vi "matrixManipulation.vi"(10 "J Index":i32, 11 "Input Array":dbl[][](array[numeric])) -> (2 "Frequency Num":string, 3 "Output Array at Frequency Num":dbl[][](array[numeric]))   [LabVIEW 2012]
uses:
  <vilib>/Analysis/Matrix/Numeric/Conversions/Array To Matrix - RA2.vi
  <vilib>/Analysis/Matrix/Numeric/Conversions/Matrix To Array - RM.vi
  <vilib>/Analysis/Matrix/NI_Matrix.lvlib
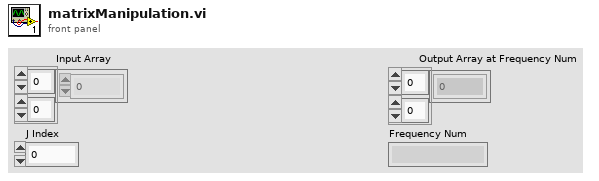
[diagram p1: front panel]
types:
  T1 = typedef "NI_Matrix.lvlib/RealMatrix.ctl" = dbl[][]
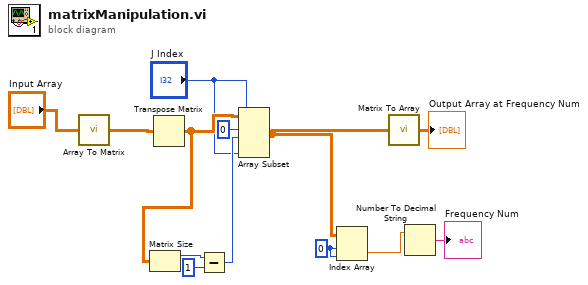
[diagram p0: block diagram]
diagram:
  w4 = 0 ("index (row)")
  n1 = call-poly <vilib>:"Array To Matrix.vi"("Real 2D Array"="Input Array") -> ("Real Matrix"=w12:T1)
  n2 = Transpose Matrix(1:w12) -> (0:w10:T1)
  n3 = Matrix Size(0:w10) -> (1:w9:i32)  [unwired: 1 out]
  n4 = Subtract(x=w9, y=1) -> (x-y=w7:i32)
  n5 = Array Subset(array=w10, index (row)=0 ("row 1"), length (row)=w7, index (col)="J Index", length (col)="J Index") -> (w1:T1)
  n6 = Index Array(array=w1, index (row)=w4, index (col)=w4) -> (element=w3:dbl)
  n7 = call-poly <vilib>:"Matrix To Array.vi"("Real Matrix"=w1) -> ("Real 2D Array"=→"Output Array at Frequency Num":dbl[][])
  n8 = Number To Decimal String(number=w3) -> (decimal integer string=→"Frequency Num":string)  [unwired: 1 in]
